vi "Get_Data.vi"(8 "error in (no error)":errorcluster caption="entrée d'erreur (pas d'erreur)", 11 "Firebase Altyor en entrée":refnum<class "Firebase Altyor.lvclass">) -> (0 "error out":errorcluster caption="sortie d'erreur", 3 "Firebase Altyor en sortie":refnum<class "Firebase Altyor.lvclass">)   [LabVIEW 2020, in "Library Instrument & Equipement.lvlib" / "Library FireBase.lvlib" / "Firebase Altyor.lvclass"]
doc: "Returns all data Use Nb_To_Read to determine the number to read\nPlease initialise the following values\n - Name BDD\n - Document\n - API Key\n - Nb To Read"
uses:
  Firebase Altyor.lvclass
  Firebase Altyor.lvclass/Firebase Altyor.ctl
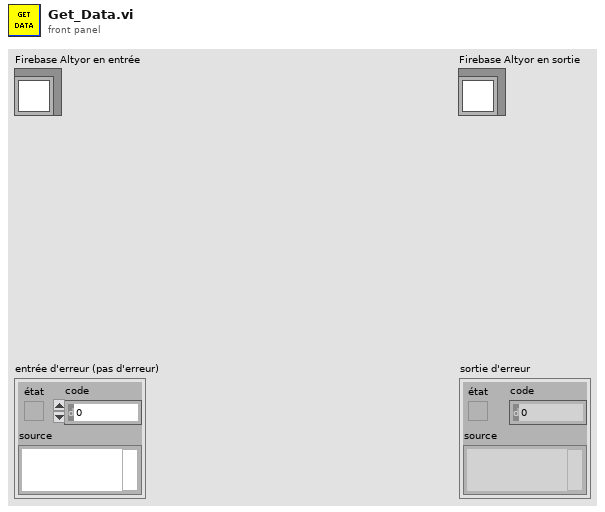
[diagram p1: front panel]
types:
  T1 = cluster{"document":cluster{"name":string, "fields":cluster{"Result":cluster{"booleanValue":bool}, "CreationDate":cluster{"timestampValue":string}, "Batch":cluster{"stringValue":string}, "SerialNumber":cluster{"stringValue":string}, "EndOfProduction":cluster{"timestampValue":string}, "FW_Version":cluster{"mapValue":cluster{"fields":cluster{"Bootloader":cluster{"mapValue":cluster{"fields":cluster{"File_Name":cluster{"stringValue":string}, "Version":cluster{"mapValue":cluster{"fields":cluster{"Major":cluster{"stringValue":string}, "Minor":cluster{"stringValue":string}}}}, "Checksum":cluster{"stringValue":string}}}}, "SoftDevice":cluster{"mapValue":cluster{"fields":cluster{"File_Name":cluster{"stringValue":string}, "Version":cluster{"mapValue":cluster{"fields":cluster{"Major":cluster{"stringValue":string}, "Minor":cluster{"stringValue":string}}}}, "Checksum":cluster{"stringValue":string}}}}, "DFU":cluster{"mapValue":cluster{"fields":cluster{"File_Name":cluster{"stringValue":string}, "Version":cluster{"mapValue":cluster{"fields":cluster{"Major":cluster{"stringValue":string}, "Minor":cluster{"stringValue":string}}}}, "Checksum":cluster{"stringValue":string}}}}}}}, "PartNumber":cluster{"stringValue":string}, "OrderNumber":cluster{"stringValue":string}, "Operator":cluster{"stringValue":string}}}}[]
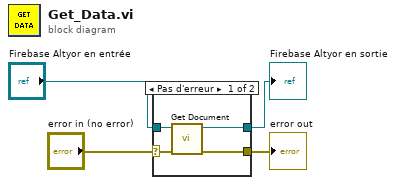
[diagram p0: block diagram]
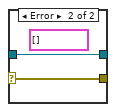
[diagram p2: hidden frame]
diagram:
  n1 = case shown="Pas d'erreur" "error in (no error)" {
    selector: "error in (no error)" -> [w6 w10]
    tunnel: [w8 w10] -> w3
    tunnel: [w7 w9] -> w1
    tunnel: "Firebase Altyor en entrée" -> [w5 w9]
    frame No Error {
      n2 = call-dynamic "Get Document.vi"("error in (no error)"=w6, "Firebase (Default) en entrée"=w5) -> ("error out"=w8:errorcluster, "Firebase (Default) en sortie"=w7:refnum<class "Firebase Altyor.lvclass">)  [unwired: 8 in]
    }
    frame Error {
      (unwired) T1 [] ("Data")
    }
  }
  "error out" <- w3
  "Firebase Altyor en sortie" <- w1
